vi "Choreo_Util_AllianceFlipPose2d.vi"(11 "Pose":T1={"TRANSLATION"={"X"=0.0, "Y"=0.0}, "ROTATION"={"VALUE"=0.0, "COS"=1.0, "SIN"=0.0}} {"ROTATION"."SIN" format="%13.4f"; "ROTATION"."COS" format="%13.4f"; "ROTATION"."VALUE" format="%13.4f"; "TRANSLATION"."Y" format="%14.3f"; "TRANSLATION"."X" format="%14.3f"}) -> (3 "FlippedPose":T1={"TRANSLATION"={"X"=0.0, "Y"=0.0}, "ROTATION"={"VALUE"=0.0, "COS"=1.0, "SIN"=0.0}} {"ROTATION"."SIN" format="%13.4f"; "ROTATION"."COS" format="%13.4f"; "ROTATION"."VALUE" format="%13.4f"; "TRANSLATION"."Y" format="%14.3f"; "TRANSLATION"."X" format="%14.3f"})   [LabVIEW 2019, in "ChoreoLib.lvlib"]
doc: "Flips a pose2d cluster.\n\nInputs: \n -- pose - pose2d - The pose to flip.\n\nOutputs:\n -- FlippedPose - pose2d - The flipped cluster"
uses:
  ChoreoLib.lvlib
  <vilib>/Rock Robotics/WPI/ThirdParty/JAS_Junk/TrajLib/TypeDef/POSE2D.ctl
  <vilib>/Rock Robotics/WPI/ThirdParty/JAS_Junk/TrajLib/TypeDef/TRANSLATION2D.ctl
  <vilib>/Rock Robotics/WPI/ThirdParty/JAS_Junk/TrajLib/TypeDef/ROTATION2D.ctl
  <vilib>/Rock Robotics/WPI/ThirdParty/JAS_Junk/TrajLib/Translation2d_GetXY.vi
  <vilib>/Rock Robotics/WPI/ThirdParty/JAS_Junk/TrajLib/Translation2d_Create.vi
  Choreo_Util_AllianceFlipX.vi
  Choreo_Util_AllianceFlipY.vi
  <vilib>/Rock Robotics/WPI/ThirdParty/JAS_Junk/TrajLib/Rotation2d_GetAngleCosSin.vi
  <vilib>/Rock Robotics/WPI/ThirdParty/JAS_Junk/TrajLib/Rotation2d_CreateXY.vi
  <vilib>/Rock Robotics/WPI/ThirdParty/JAS_Junk/TrajLib/Util_CalcDist.vi
  Choreo_Choreo_Globals.vi
  <vilib>/Rock Robotics/WPI/ThirdParty/JAS_Junk/TrajLib/Trajectory_Library.lvlib
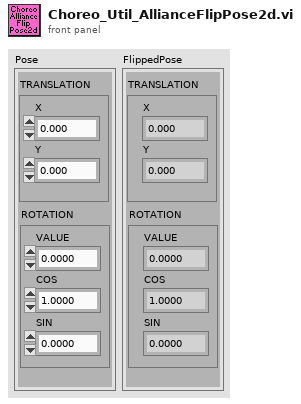
[diagram p1: front panel]
types:
  T1 = typedef "Trajectory_Library.lvlib/POSE2D.ctl" = cluster{"TRANSLATION":T2, "ROTATION":T3}
  T2 = typedef "Trajectory_Library.lvlib/TRANSLATION2D.ctl" = cluster{"X":dbl, "Y":dbl}
  T3 = typedef "Trajectory_Library.lvlib/ROTATION2D.ctl" = cluster{"VALUE":dbl, "COS":dbl, "SIN":dbl}
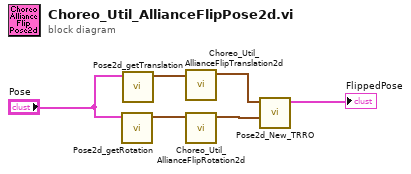
[diagram p0: block diagram]
diagram:
  n1 = call <vilib>:"Pose2d_getRotation.vi"("in POSE"="Pose") -> ("out ROTATION"=w4:T3)  [unwired: 10 in]
  n2 = call <vilib>:"Pose2d_getTranslation.vi"("in POSE"="Pose") -> ("outTRANSLATION"=w5:T2)  [unwired: 10 in]
  n3 = call "Choreo_Util_AllianceFlipTranslation2d.vi"("Translation"=w5) -> ("FlippedTranslation"=w3:T2)  [unwired: 10 in]
  n4 = call "Choreo_Util_AllianceFlipRotation2d.vi"("Rotation"=w4) -> ("FlippedRotation"=w2:T3)  [unwired: 10 in]
  n5 = call <vilib>:"Pose2d_New_TRRO.vi"("ROTATION"=w2, "TRANSLATION"=w3) -> ("outPOSE"=→"FlippedPose":T1)  [unwired: 9 in]
